vi "Arm.vi"(4 "Request type":T1=enum."User command", 6 "Init work":bool, 7 "Update period":dbl, 8 "error in (no error)":errorcluster, 9 "Last request":bool, 10 "Requester":string, 11 "Pulse Recorder Actor in":refnum<class "Pulse Recorder Actor.lvclass">) -> (0 "error out":errorcluster, 3 "Pulse Recorder Actor out":refnum<class "Pulse Recorder Actor.lvclass">)   [LabVIEW 2021, in "Pulse Recorder Actor.lvclass"]
uses:
  Pulse Recorder Actor.lvclass
  Controllers/Process Controller/Request type.ctl
  Read Pulse driver.vi
  Write Pulse driver.vi
  NHMFL_Core/Libraries/Instruments/Pulse Driver/Pulse Driver.lvclass
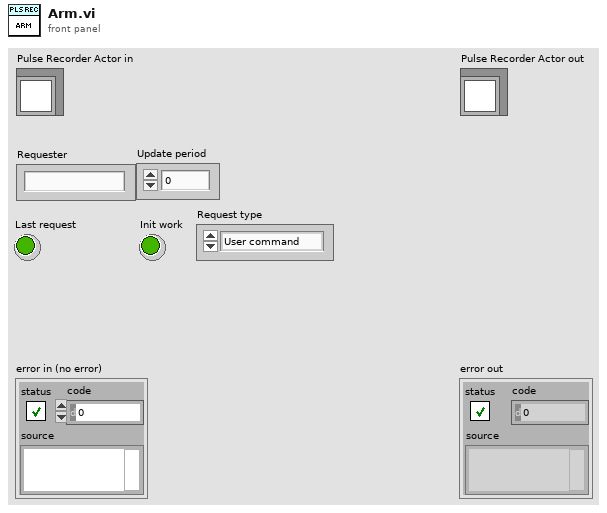
[diagram p1: front panel]
types:
  T1 = typedef "Request type.ctl" = enum16{"Process complete", "User command", "Auto-restart", "Error"}
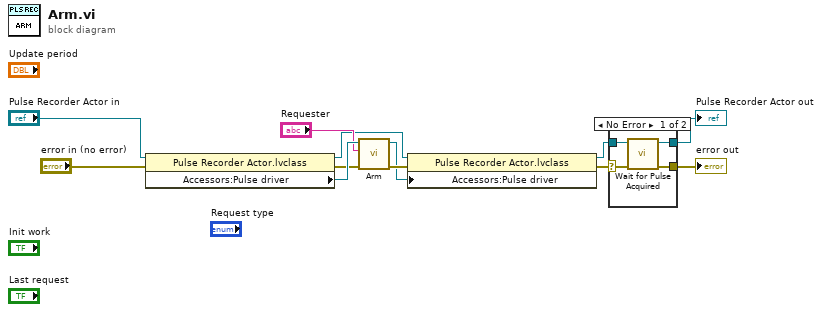
[diagram p0: block diagram]
diagram:
  n1 = property class="Pulse Recorder Actor.lvclass"(reference="Pulse Recorder Actor in", error in="error in (no error)") -> (reference out=w6:refnum<class "Pulse Recorder Actor.lvclass">, error out=w10:errorcluster, "Accessors:Pulse driver"=w11:refnum<class "Pulse Driver.lvclass">)
  n2 = call-dynamic "Arm.vi"("error in (no error)"=w10, "Controller name"="Requester", "Pulse Driver in"=w11) -> ("error out"=w8:errorcluster, "Pulse Driver out"=w7:refnum<class "Pulse Driver.lvclass">)  [unwired: 7 in]
  n3 = property class="Pulse Recorder Actor.lvclass"(reference=w6, error in=w8, "Accessors:Pulse driver"=w7) -> (reference out=w4:refnum<class "Pulse Recorder Actor.lvclass">, error out=w5:errorcluster)
  n4 = case shown="No Error" w5 {
    selector: w5 -> [w16 w17]
    tunnel: w4 -> [w15 w18]
    tunnel: [w14 w18] -> w3
    tunnel: [w13 w17] -> w1
    frame No Error {
      n5 = call-dynamic "Wait for Pulse Acquired.vi"("error in (no error)"=w16, "Pulse Recorder Actor in"=w15) -> ("error out"=w13:errorcluster, "Pulse Recorder Actor out"=w14:refnum<class "Pulse Recorder Actor.lvclass">)  [unwired: 8 in]
    }
    frame Error {
    }
  }
  "error out" <- w1
  "Pulse Recorder Actor out" <- w3
